vi "Teleop.vi"(10 "Match Info":T1={"Autonomous Elapsed Seconds"=0.0, "TeleOp Elapsed Seconds"=0.0, "Disabled Elapsed Seconds"=0.0, "Visited Autonomous"=FALSE, "Visited TeleOp"=FALSE, "Visited Disabled"=FALSE, "Autonomous Settings"={"Autonomous Style"=enum."Independent", "VI Refnum"=refnum}}, 11 "Call Context":T2) -> ()   [LabVIEW 2016]
doc: "This VI is called for each enabled TeleOp packet received from the DS. It is typically used to read from joysticks and other inputs and update I/O or setpoints for timed control loops. It should complete and return within 20 milliseconds or risk missing DS packets."
uses:
  <vilib>/Rock Robotics/WPI/DriverStation/WPI_DriverStationDerivedRobotMode.ctl
  <vilib>/Rock Robotics/WPI/DriverStation/WPI_DriverStationMatch Info.ctl
  <vilib>/Rock Robotics/WPI/Solenoid/WPI_SolenoidValue.ctl
  <vilib>/Rock Robotics/WPI/Utilities/WPI_GetSetVariantRefNum.vi
  <vilib>/Rock Robotics/Network Tables/NT Write Boolean Array.vi
  <vilib>/Rock Robotics/Network Tables/NT Write Numeric Array.vi
  Winch/Implementation/Winch Globals.vi
  NavX/NavX Global.vi
  <vilib>/Rock Robotics/WPI/Solenoid/WPI_SolenoidSetEnum.vi
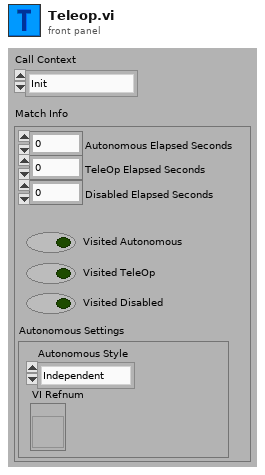
[diagram p1: front panel]
types:
  T1 = typedef "WPI_DriverStationMatch Info.ctl" = cluster{"Autonomous Elapsed Seconds":dbl, "TeleOp Elapsed Seconds":dbl, "Disabled Elapsed Seconds":dbl, "Visited Autonomous":bool, "Visited TeleOp":bool, "Visited Disabled":bool, "Autonomous Settings":cluster{"Autonomous Style":enum16{"Iterative", "Independent"}, "VI Refnum":refnum<vi>}}
  T2 = typedef "WPI_DriverStationDerivedRobotMode.ctl" = enum16{"Init", "Execute", "Stop"}
  T3 = typedef "WPI_SolenoidValue.ctl" = enum16{"Off", "On", "Forward", "Reverse"}
  T4 = typedef "WPI_JoystickDevRef.ctl" = cluster{"Device":T5}
  T5 = typedef "WPI_JoystickDeviceEnum.ctl" = enum16{"USB 0", "USB 1", "USB 2", "USB 3", "USB 4", "USB 5"}
  T6 = typedef "WPI_ServoDeviceRef.ctl" = cluster{"DeviceStatus":errorcluster, "PWM Channel":T7, "DeadBand":T8}
  T7 = typedef "FPGA_DIOPWMChannel.ctl" = enum8{"PWM 0", "PWM 1", "PWM 2", "PWM 3", "PWM 4", "PWM 5", "PWM 6", "PWM 7", "PWM 8", "PWM 9", "PWM MXP 0", "PWM MXP 1", "PWM MXP 2", "PWM MXP 3", "PWM MXP 4", "PWM MXP 5", "PWM MXP 6", "PWM MXP 7", "PWM MXP 8", "PWM MXP 9", "Invalid"}
  T8 = typedef "WPI_PWMDeadband.ctl" = cluster{"Name":string, "maxPositivePwm":i32, "minPositivePwm":i32, "centerPwm":i32, "maxNegativePwm":i32, "minNegativePwm":i32, "angularRange":u16}
  T9 = typedef "WPI_SolenoidDevRef.ctl" = cluster{"DevStatus":errorcluster, "Pneumatics Control Module":u8, "Forward Solenoid Channel":T10, "Reverse Solenoid Channel":T10}
  T10 = typedef "WPI_SolenoidChannel.ctl" = enum8{"Solenoid 0", "Solenoid 1", "Solenoid 2", "Solenoid 3", "Solenoid 4", "Solenoid 5", "Solenoid 6", "Solenoid 7", "Invalid"}
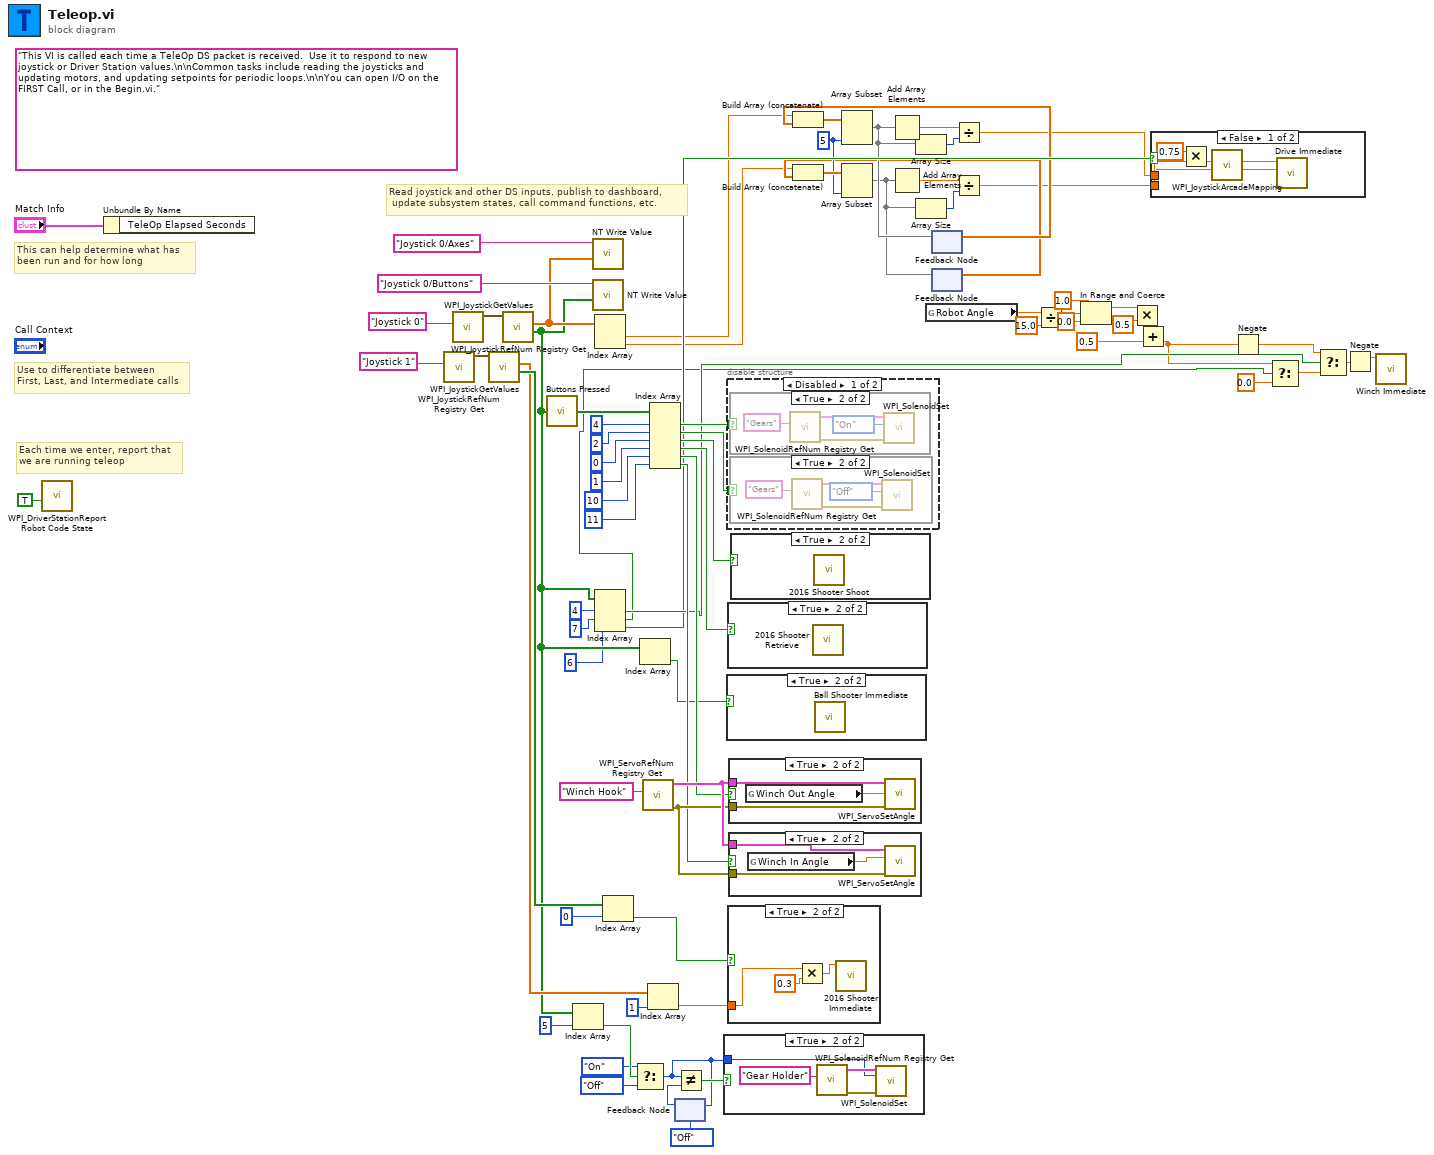
[diagram p0: block diagram]
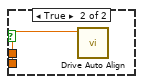
[diagram p5: hidden frame]
diagram:
  w10 = 5 ("length")
  (unwired) "This VI is called each time a TeleOp DS packet is received.  Use it to respond to new joystick or Driver Station values.\n\nCommon tasks include reading the joysticks and updating motors, and updating setpoints for periodic loops.\n\nYou can open I/O on the FIRST Call, or in the Begin.vi."
  # "Read joystick and other DS inputs, publish to dashboard,\n update subsystem states, call command functions, etc."
  # "Each time we enter, report that\nwe are running teleop"
  # "Use to differentiate between\nFirst, Last, and Intermediate calls"
  # "This can help determine what has\nbeen run and for how long"
  n1 = call <vilib>:"WPI_DriverStationReport Robot Code State.vi"("TeleOp"=TRUE ("Autonomous")) -> ()  [unwired: 10 in, 1 out]
  n2 = Unbundle By Name("Match Info") -> ()  [unwired: 1 out]
  n3 = call <vilib>:"WPI_JoystickRefNum Registry Get.vi"("refnum name"="Joystick 1") -> ("JoystickDevRef"=w55:T4)  [unwired: 1 in, 9 out]
  n4 = call <vilib>:"WPI_JoystickRefNum Registry Get.vi"("refnum name"="Joystick 0") -> ("JoystickDevRef"=w74:T4)  [unwired: 1 in, 9 out]
  n5 = call <vilib>:"WPI_JoystickGetValues.vi"("JoystickDevRef"=w55) -> ("Buttons"=w53:bool[], "Axes"=w50:dbl[])  [unwired: 6 in, 3 out]
  n6 = call <vilib>:"WPI_JoystickGetValues.vi"("JoystickDevRef"=w74) -> ("Buttons"=w36:bool[], "Axes"=w72:dbl[])  [unwired: 6 in, 3 out]
  n7 = call "Buttons Pressed.vi"("Button Values"=w36) -> ("Button Presses"=w38:bool[])
  n8 = Index Array(array=w36, index=5) -> (element=w65:bool)
  n9 = call-poly <vilib>:"NT Write Value.vi"("Numeric Array"=w72, "Name"="Joystick 0/Axes") -> ()  [unwired: 9 in, 1 out]
  n10 = call-poly <vilib>:"NT Write Value.vi"("Boolean Array"=w36, "Name"="Joystick 0/Buttons") -> ()  [unwired: 9 in, 1 out]
  n11 = Index Array(array=w72) -> (element #1=w3:dbl, element #2=w4:dbl)  [unwired: 2 in]
  n12 = Index Array(array=w36, index #1=4 ("index"), index #2=7 ("index"), index #3=6 ("index")) -> (element #1=w33:bool, element #2=w17:bool, element #3=w28:bool)
  n13 = Index Array(array=w53, index=0) -> (element=w52:bool)
  n14 = Select(t=WPI_SolenoidValue."On" ("Value"), s=w65, f=WPI_SolenoidValue."Off" ("Value")) -> (s? t:f=w60:T3)
  n15 = Index Array(array=w36) -> (element=w37:bool)  [unwired: 1 in]
  n16 = call <vilib>:"WPI_ServoRefNum Registry Get.vi"("refnum name"="Winch Hook") -> ("error out"=w56:errorcluster, "ServoDeviceRef"=w57:T6)  [unwired: 9 in]
  n17 = Index Array(array=w50, index=1) -> (element=w48:dbl)
  n18 = Index Array(array=w38, index #1=4 ("index"), index #2=2 ("index"), index #3=0 ("index"), index #4=1 ("index"), index #5=10 ("index"), index #6=11 ("index")) -> (element #1=w68:bool, element #2=w67:bool, element #3=w46:bool, element #4=w44:bool, element #5=w41:bool, element #6=w40:bool)
  n19 = feedback-in #1(w60) -> ()
  n20 = feedback #1(WPI_SolenoidValue."Off" ("Value")) -> (w61:T3)
  n21 = Not Equal?(x=w60, y=w61) -> (x != y?=w62:bool)
  n22 = case shown="True" w62 {
    tunnel: w60 -> [_ w78]
    frame False {
    }
    frame True {
      n23 = call <vilib>:"WPI_SolenoidRefNum Registry Get.vi"("refnum name"="Gear Holder") -> ("error out"=w79:errorcluster, "SolenoidDevRef"=w80:T9)  [unwired: 9 in]
      n24 = call-poly <vilib>:"WPI_SolenoidSet.vi"("error in (no error)"=w79, "Value"=w78, "SolenoidDevRef"=w80) -> ()  [unwired: 7 in, 2 out]
    }
  }
  n25 = case shown="True" w37 {
    frame False {
    }
    frame True {
      n26 = call "Ball Shooter Immediate.vi"() -> ()  [unwired: 11 in, 1 out]
    }
  }
  n27 = disable-structure shown="Disabled" {
    disable-tunnel: w68 -> [w83 _]
    disable-tunnel: w67 -> [w82 _]
    frame Disabled {
      n28 = case shown="True" w83 {
        frame False {
        }
        frame True {
          n29 = call <vilib>:"WPI_SolenoidRefNum Registry Get.vi"("refnum name"="Gears") -> ("error out"=w89:errorcluster, "SolenoidDevRef"=w90:T9)  [unwired: 9 in]
          n30 = call-poly <vilib>:"WPI_SolenoidSet.vi"("error in (no error)"=w89, "Value"=WPI_SolenoidValue."On", "SolenoidDevRef"=w90) -> ()  [unwired: 7 in, 2 out]
        }
      }
      n31 = case shown="True" w82 {
        frame False {
        }
        frame True {
          n32 = call <vilib>:"WPI_SolenoidRefNum Registry Get.vi"("refnum name"="Gears") -> ("error out"=w85:errorcluster, "SolenoidDevRef"=w86:T9)  [unwired: 9 in]
          n33 = call-poly <vilib>:"WPI_SolenoidSet.vi"("error in (no error)"=w85, "Value"=WPI_SolenoidValue."Off", "SolenoidDevRef"=w86) -> ()  [unwired: 7 in, 2 out]
        }
      }
    }
    frame Enabled {
    }
  }
  n34 = case shown="True" w44 {
    frame False {
    }
    frame True {
      n35 = call "2016 Shooter Retrieve.vi"() -> ()  [unwired: 11 in, 1 out]
    }
  }
  n36 = case shown="True" w52 {
    tunnel: w48 -> [_ w92]
    frame False {
    }
    frame True {
      n37 = Multiply(x=w92, y=0.3) -> (x*y=w93:dbl)
      n38 = call "2016 Shooter Immediate.vi"("Setpoint"=w93) -> ()  [unwired: 10 in, 1 out]
    }
  }
  n39 = case shown="True" w41 {
    tunnel: w56 -> [_ w97]
    tunnel: w57 -> [_ w96]
    frame False {
    }
    frame True {
      n40 = global read "Winch Globals.vi" "Winch Out Angle"() -> (w95:dbl)
      n41 = call <vilib>:"WPI_ServoSetAngle.vi"("error in (no error)"=w97, "Angle"=w95, "ServoDeviceRef"=w96) -> ()  [unwired: 7 in, 2 out]
    }
  }
  n42 = case shown="True" w40 {
    tunnel: w56 -> [_ w100]
    tunnel: w57 -> [_ w99]
    frame False {
    }
    frame True {
      n43 = global read "Winch Globals.vi" "Winch In Angle"() -> (w98:dbl)
      n44 = call <vilib>:"WPI_ServoSetAngle.vi"("error in (no error)"=w100, "Angle"=w98, "ServoDeviceRef"=w99) -> ()  [unwired: 7 in, 2 out]
    }
  }
  n45 = case shown="True" w46 {
    frame False {
    }
    frame True {
      n46 = call "2016 Shooter Shoot.vi"() -> ()  [unwired: 11 in, 1 out]
    }
  }
  n47 = global read "NavX Global.vi" "Robot Angle"() -> (w27:dbl)
  n48 = feedback #2() -> (w6:dbl[])  [unwired: 1 in]
  n49 = Build Array (concatenate)(w3, w6) -> (w15:dbl[])
  n50 = Array Subset(array=w15, length=w10) -> (w13:dbl[])  [unwired: 1 in]
  n51 = Add Array Elements(numeric array=w13) -> (sum=w14:dbl)
  n52 = Array Size(array=w13) -> (size(s)=w12:i32)
  n53 = feedback-in #2(w13) -> ()
  n54 = feedback #3() -> (w5:dbl[])  [unwired: 1 in]
  n55 = Build Array (concatenate)(w4, w5) -> (w11:dbl[])
  n56 = Array Subset(array=w11, length=w10) -> (w9:dbl[])  [unwired: 1 in]
  n57 = Add Array Elements(numeric array=w9) -> (sum=w8:dbl)
  n58 = Array Size(array=w9) -> (size(s)=w7:i32)
  n59 = feedback-in #3(w9) -> ()
  n60 = Divide(x=w14, y=w12) -> (x/y=w2:dbl)
  n61 = Divide(x=w8, y=w7) -> (x/y=w1:dbl)
  n62 = Divide(x=w27, y=15.0) -> (x/y=w25:dbl)
  n63 = In Range and Coerce(upper limit=1.0, x=w25, lower limit=0.0) -> (coerced(x)=w22:dbl)  [unwired: 1 out]
  n64 = Multiply(x=w22, y=0.5) -> (x*y=w19:dbl)
  n65 = Add(x=w19, y=0.5) -> (x+y=w20:dbl)
  n66 = case shown="False" w28 {
    tunnel: w2 -> [w104 _]
    tunnel: w1 -> [w103 w107]
    frame False {
      n67 = Multiply(x=0.75, y=w104) -> (x*y=w102:dbl)
      n68 = call <vilib>:"WPI_JoystickArcadeMapping.vi"("Y axis value"=w103, "X axis value"=w102) -> ("Right Motor Value"=w106:dbl, "Left Motor Value"=w105:dbl)  [unwired: 8 in]
      n69 = call "Drive Immediate.vi"("Right Setpoint"=w106, "Left Setpoint"=w105) -> ()  [unwired: 9 in, 1 out]
    }
    frame True {
      n70 = call "Drive Auto Align.vi"("Left Setpoint"=w107) -> ()  [unwired: 9 in, 2 out]
    }
  }
  n71 = Negate(x=w20) -> (-x=w31:dbl)
  n72 = Select(t=w20, s=w17, f=0.0) -> (s? t:f=w34:dbl)
  n73 = Select(t=w31, s=w33, f=w34) -> (s? t:f=w18:dbl)
  n74 = Negate(x=w18) -> (-x=w16:dbl)
  n75 = call "Winch Immediate.vi"("Setpoint"=w16) -> ()  [unwired: 10 in, 1 out]
